vi "Set Self Attributes.vi"(10 "Self Attributes":T1, 11 "Base Sender in":refnum<class "Base Sender.lvclass">) -> (3 "Base Sender out":refnum<class "Base Sender.lvclass">)   [LabVIEW 2020, in "jettl.lvlib" / "Sender.lvlib" / "Base Sender.lvclass"]
uses:
  Base Sender.lvclass
  Msg/Msg.lvclass
  Actor/Implemented Msgs.ctl
  Actor/Actor.lvlib
  Actor/Attributes.ctl
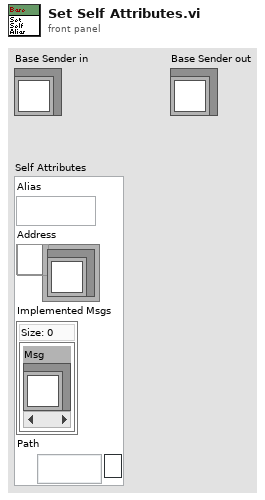
[diagram p1: front panel]
types:
  T1 = typedef "jettl.lvlib/Actor.lvlib/Attributes.ctl" = cluster{"Alias":string, "Address":refnum<user-event>, "Implemented Msgs":T2, "Path":path}
  T2 = typedef "jettl.lvlib/Actor.lvlib/Implemented Msgs.ctl" = set{refnum<class "Msg.lvclass">}
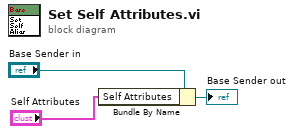
[diagram p0: block diagram]
diagram:
  n1 = Bundle By Name(cluster="Base Sender in", "Self Attributes"="Self Attributes") -> (→"Base Sender out":refnum<class "Base Sender.lvclass">)
